vi "Write Name.vi"(8 "error in (no error)":errorcluster, 10 "Name":string, 11 "Test Group in":refnum<class "Test Group.lvclass">) -> (0 "error out":errorcluster, 3 "Test Group out":refnum<class "Test Group.lvclass">)   [LabVIEW 2018, in "Test Number and Bin Generator.lvlib" / "Test Group.lvclass"]
uses:
  Test Group.lvclass
  Test Group.lvclass/Test Group.ctl
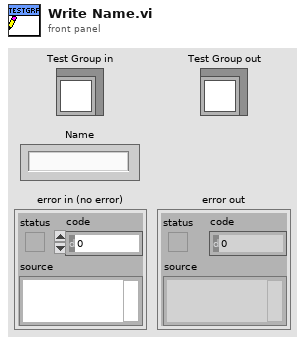
[diagram p1: front panel]
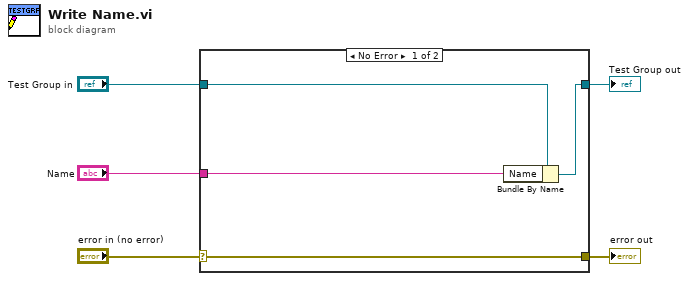
[diagram p0: block diagram]
diagram:
  n1 = case shown="No Error" "error in (no error)" {
    selector: "error in (no error)" -> [w9 w10]
    tunnel: [w9 w10] -> w4
    tunnel: [w7 w11] -> w2
    tunnel: "Test Group in" -> [w8 w11]
    tunnel: "Name" -> [w6 _]
    frame No Error {
      n2 = Bundle By Name(cluster=w8, "Name"=w6) -> (w7:refnum<class "Test Group.lvclass">)
    }
    frame Error {
    }
  }
  "error out" <- w4
  "Test Group out" <- w2
